vi "File_Array_test code.vi"() -> ()   [LabVIEW 2015]
panel:
  out "Waveform Graph":dbl[](graph)
  in  "stop":bool
  in  "Boolean":bool
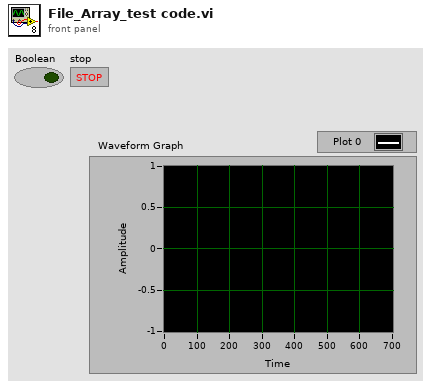
[diagram p1: front panel]
types:
  T1 = enum16{"open", "replace", "create", "open or create", "replace or create", "replace or create with confirmation"}
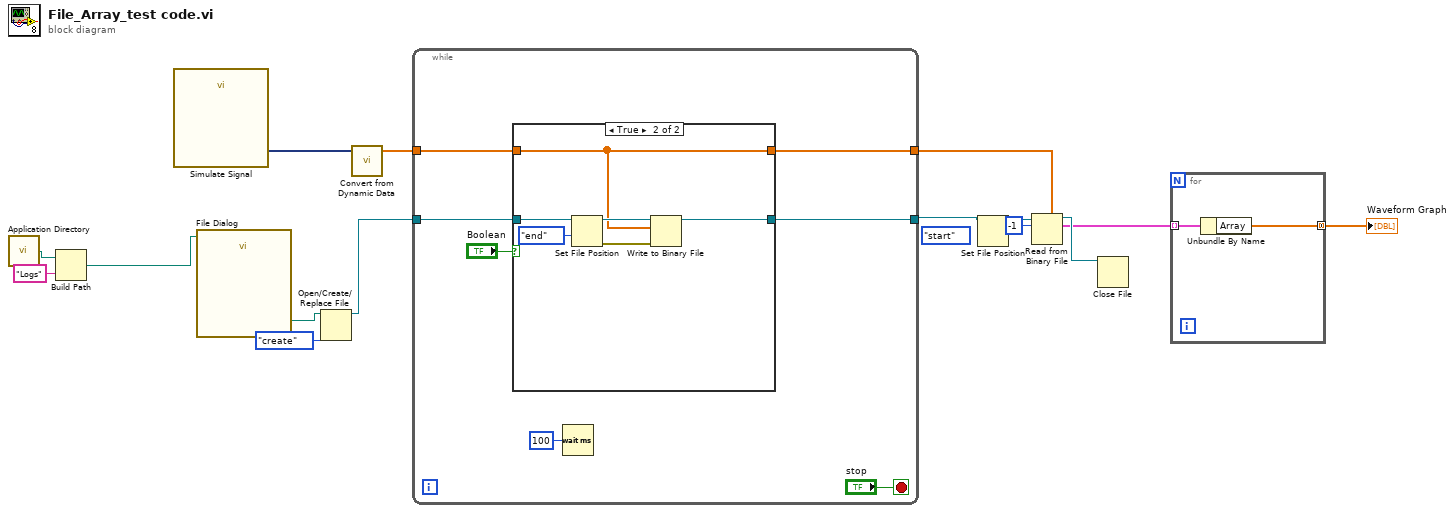
[diagram p0: block diagram]
diagram:
  (unwired) enum16{"start", "end", "current"}."start" ("from (0:start)")
  n1 = call <vilib>:"Application Directory.vi"() -> ("Application Directory"=w15:path)
  n2 = Build Path(base path=w15, name or relative path="Logs") -> (appended path=w13:path)
  n3 = call "Simulate Signal"() -> ("Sine"=w10:dynamicdata)  [unwired: 14 in, 1 out]
  n4 = call "File Dialog"("start path"=w13) -> ("selected path"=w12:path)  [unwired: 11 in, 3 out]
  n5 = Open/Create/Replace File(file path (use dialog)=w12, operation (0:open)=T1."create") -> (refnum out=w11:refnum<file>)  [unwired: 4 in, 2 out]
  n6 = call "Convert from Dynamic Data"("Dynamic Data Type"=w10) -> ("Array"=w9:dbl[])  [unwired: 3 in]
  n7 = while {
    tunnel: w11 -> [w22]
    tunnel: w9 -> [w18]
    tunnel: [w17] -> w5
    tunnel: [w16] -> w8
    stop <- "stop" stop-if-true
    n8 = case shown="True" "Boolean" {
      tunnel: w22 -> [w24 w27]
      tunnel: w18 -> [w23 w25]
      tunnel: [w24 w26] -> w17
      tunnel: [w23 w25] -> w16
      frame False {
      }
      frame True {
        n9 = Set File Position(refnum=w27, from (0:start)=enum16{"start", "end", "current"}."end") -> (refnum out=w29:refnum<file>, error out=w28:errorcluster)  [unwired: 2 in]
        n10 = Write to Binary File(file (use dialog)=w29, data=w25, error in=w28) -> (refnum out=w26:refnum<file>)  [unwired: 3 in, 2 out]
      }
    }
    n11 = Wait (ms)(milliseconds to wait=u32 100) -> ()  [unwired: 1 out]
  }
  n12 = Set File Position(refnum=w5) -> (refnum out=w4:refnum<file>)  [unwired: 3 in, 1 out]
  n13 = Read from Binary File(5:w8, 10:-1 ("count (1)"), 11:w4) -> (2:w2:cluster{"Array":dbl[]}[], 3:w6:refnum<file>)  [unwired: 3 in, 2 out]
  n14 = Close File(refnum=w6) -> ()  [unwired: 1 in, 2 out]
  n15 = for {
    tunnel: w2 -> [w32] mode=indexing
    tunnel: [w31] -> w1 mode=concatenating
    n16 = Unbundle By Name(w32) -> ("Array"=w31:dbl[])
  }
  "Waveform Graph" <- w1
